vi "TDC_getDeviceParams.vi"(8 "Error In":errorcluster) -> (0 "Error Out":errorcluster, 1 "Exposure Time [ms]":i32, 2 "Coincidence Window [ps]":i32)   [LabVIEW 2011]
uses:
  tdcbase.dll
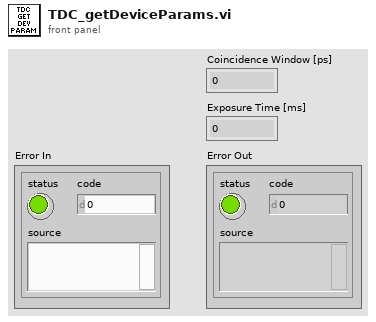
[diagram p1: front panel]
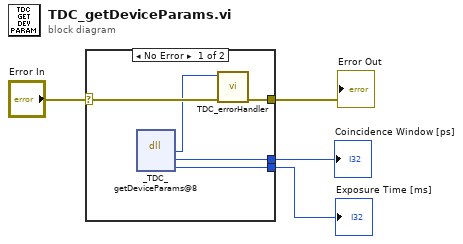
[diagram p0: block diagram]
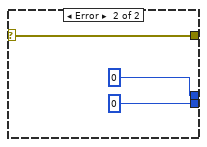
[diagram p2: hidden frame]
diagram:
  n1 = case shown="No Error" "Error In" {
    selector: "Error In" -> [w7 w12]
    tunnel: [w6 w12] -> w3
    tunnel: [w9 0] -> w2
    tunnel: [w8 0] -> w1
    frame No Error {
      n2 = dll-call lib="X:/tdcbase.dll" fn="_TDC_getDeviceParams@8"() -> ("return type"=w5:i32, "coincWin"=w9:i32, "expTime"=w8:i32)  [unwired: 5 in, 2 out]
      n3 = call "TDC_errorHandler.vi"("Error In"=w7, "TDC Return Code"=w5) -> ("Error Out"=w6:errorcluster)  [unwired: 9 in]
    }
    frame Error {
    }
  }
  "Error Out" <- w3
  "Coincidence Window [ps]" <- w2
  "Exposure Time [ms]" <- w1
